vi "UPS_Monitor.vi"() -> ()   [LabVIEW 2023]
doc: "This is the Main VI that performs the UPS and capture data from DAQ and simulate the UPS"
uses:
  Controls/Acquired_Datactl_Display.ctl
  Controls/Queue_Operation_Select.ctl
  Controls/UPS_Data.ctl
  Controls/Acquired_Data.ctl
  Controls/State_and_Data.ctl
  Controls/Notifier_Operation_Select.ctl
  Controls/File_Operation_Select.ctl
  Controls/Error_Data.ctl
panel:
  out "Error_Out":errorcluster
  in  "Error_In":errorcluster
  in  "Tab Control":enum32{"PARAMETER", "DETAILS"}(tab)
  out "ACQUIRED_DATA":T1 {"Power_Consumption" scale=0.0..10.0; "Battery_Power" scale=0.0..100.0}
  out "Low_Power_Indicator":bool caption="Low Power Indicator"
  out "Waveform Graph":dbl[][](graph)
  in  "Record":bool
  in  "Stop":bool
  in  "Pause":bool
  in  "Start":bool
  # "UPS Monitor"
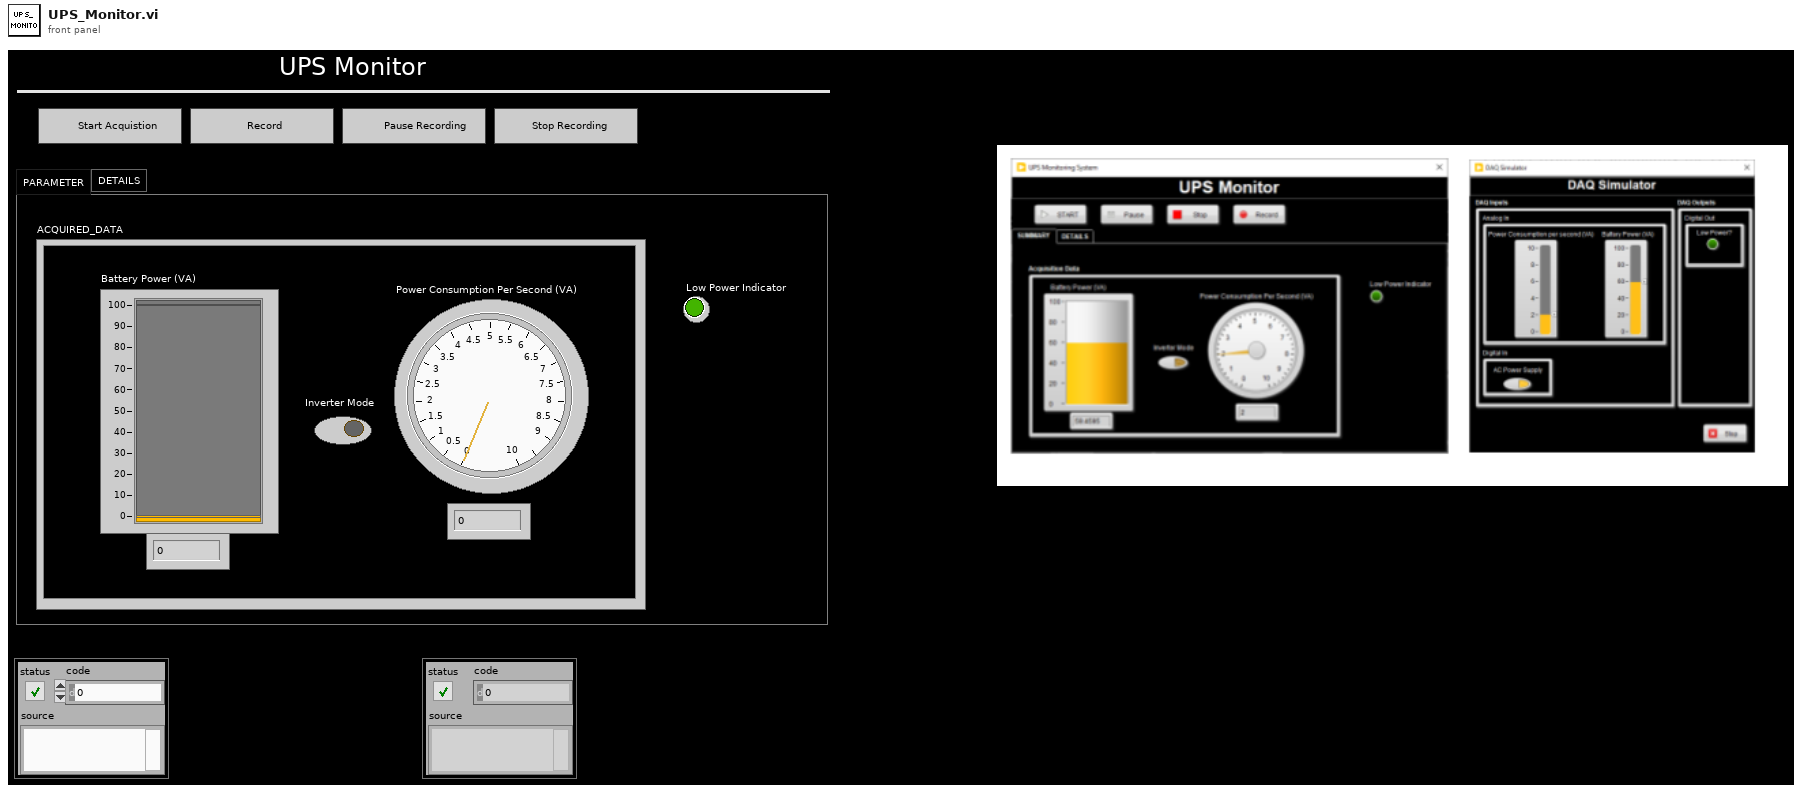
[diagram p1: front panel]
types:
  T1 = typedef "Acquired_Datactl_Display.ctl" = cluster{"Battery_Power":dbl, "Power_Consumption":dbl, "Inverter_Mode":bool}
  T2 = typedef "File_Operation_Select.ctl" = enum16{"Open", "Write", "Read", "Close"}
  T3 = typedef "Queue_Operation_Select.ctl" = enum16{"Obtain_Queue", "Enqueue", "Enqueue_First", "Enqueue_N", "Lossy_Enqueue", "Preview", "Queue_Status", "Dequeue", "Flush", "Release_Queue"}
  T4 = typedef "Notifier_Operation_Select.ctl" = enum16{"Obtain_Notifier", "Send_Notification", "Get_Notifier_Status", "Release_Notifier"}
  T5 = typedef "State_and_Data.ctl" = cluster{"State":string, "Data":variant}
  T6 = typedef "UPS_Data.ctl" = cluster{"ACQUIRED_DATA":T7, "Start":bool, "Pause":bool, "Record":bool, "Low_Power":bool, "Power_and_Power_Consumed":dbl[][], "State_and_Data_In":T5, "File_Path":path, "Application_Directory":path, "Record_Select":enum8{"Enabled", "Disabled", "Disabled and Grayed Out"}, "Stop_Select":enum8{"Enabled", "Disabled", "Disabled and Grayed Out"}}
  T7 = typedef "Acquired_Data.ctl" = cluster{"Battery_Power":dbl, "Power_Consumption":dbl, "Inverter_Mode":bool}
  T8 = enum8{"Enabled", "Disabled", "Disabled and Grayed Out"}
  T9 = typedef "Error_Data.ctl" = cluster{"Module_Name":string, "Error":errorcluster}
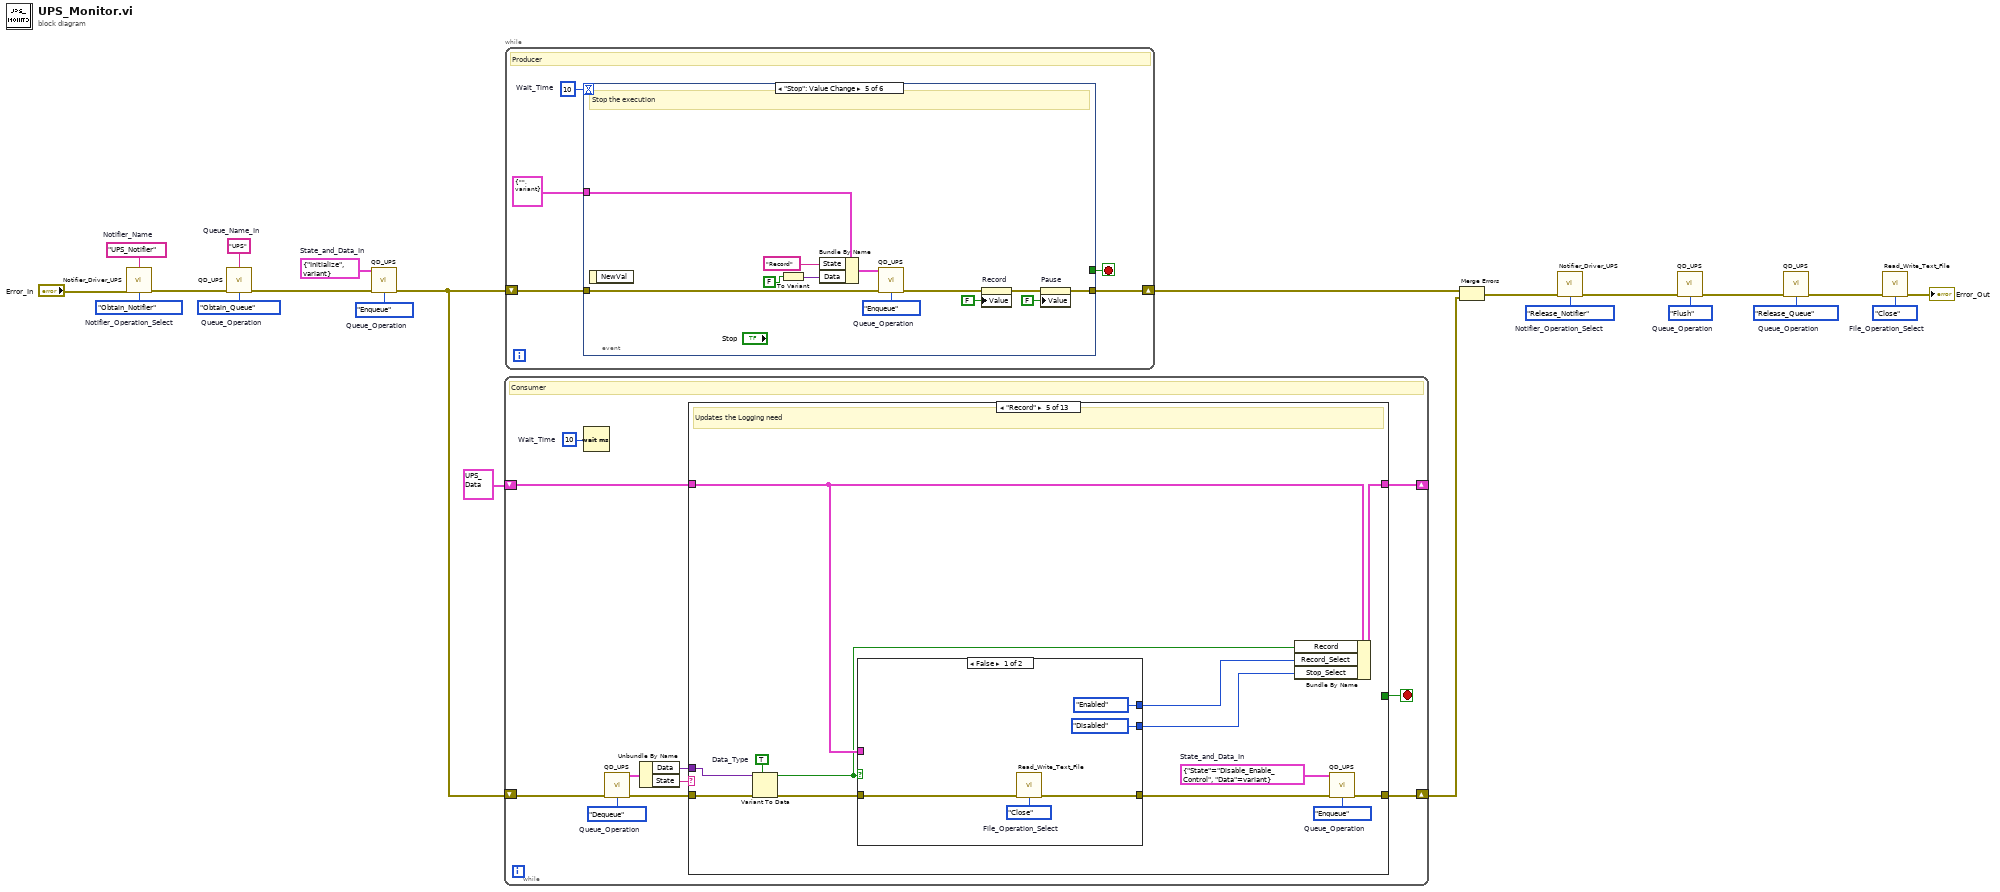
[diagram p0: block diagram]
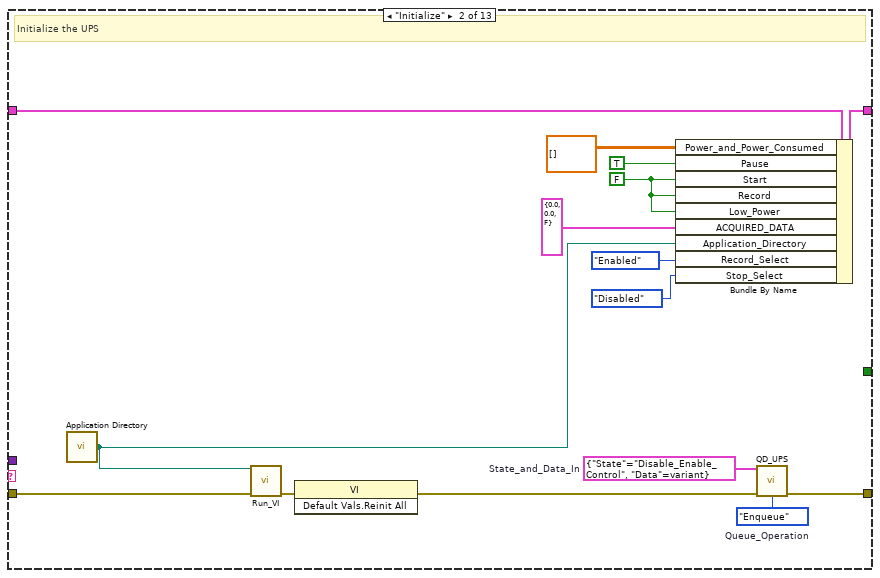
[diagram p3: hidden frame]
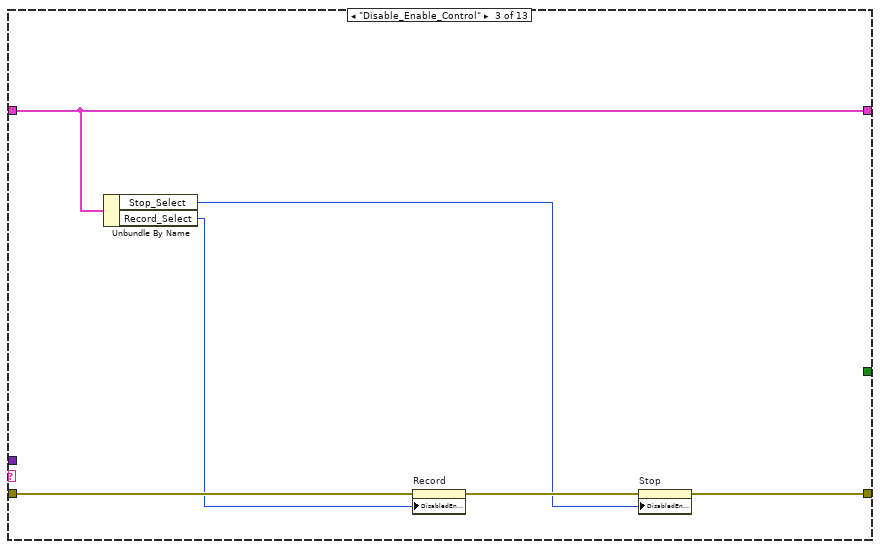
[diagram p4: hidden frame]
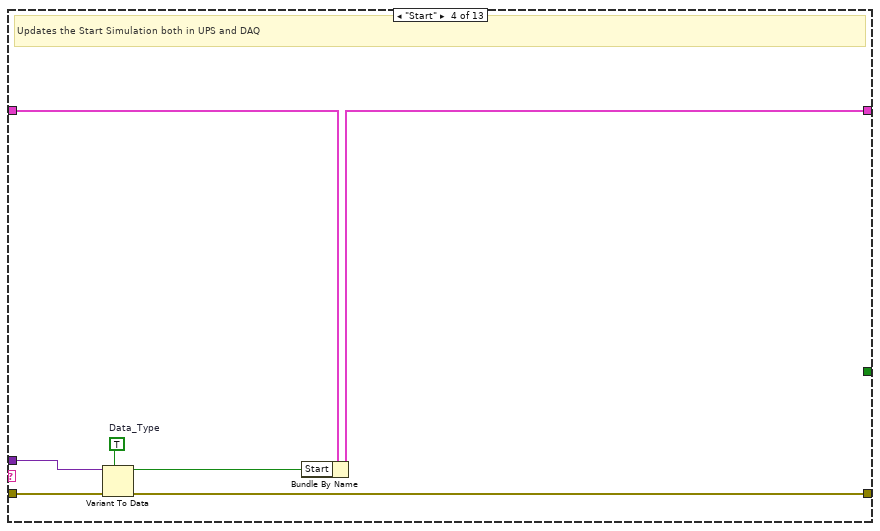
[diagram p5: hidden frame]
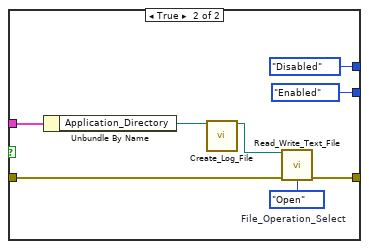
[diagram p6: hidden frame]
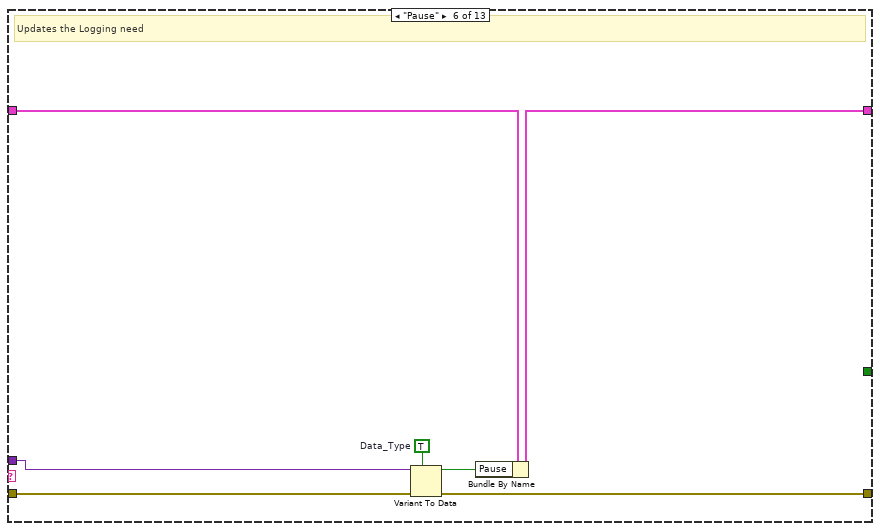
[diagram p7: hidden frame]
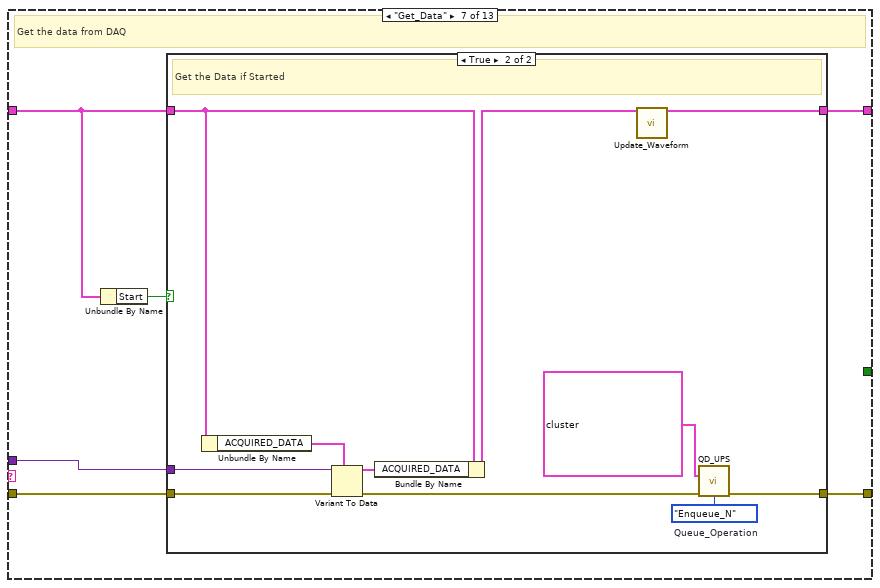
[diagram p8: hidden frame]
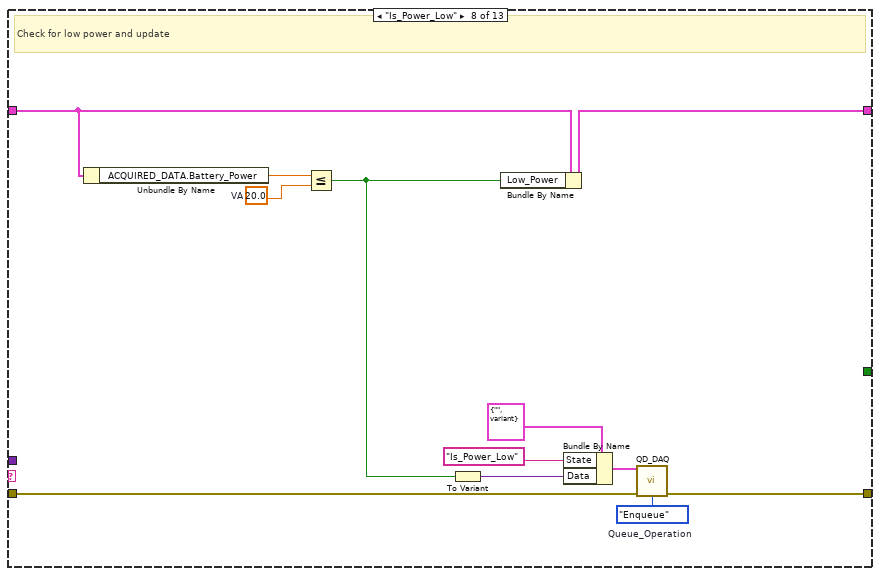
[diagram p10: hidden frame]
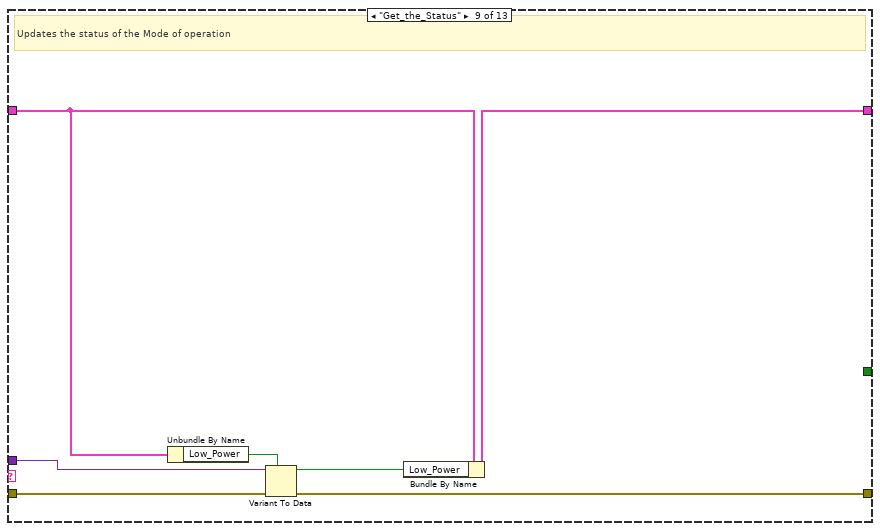
[diagram p11: hidden frame]
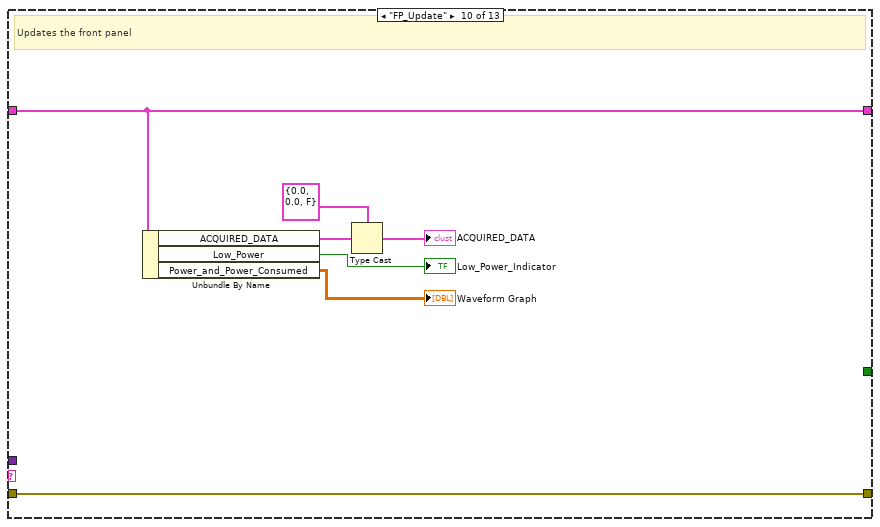
[diagram p12: hidden frame]
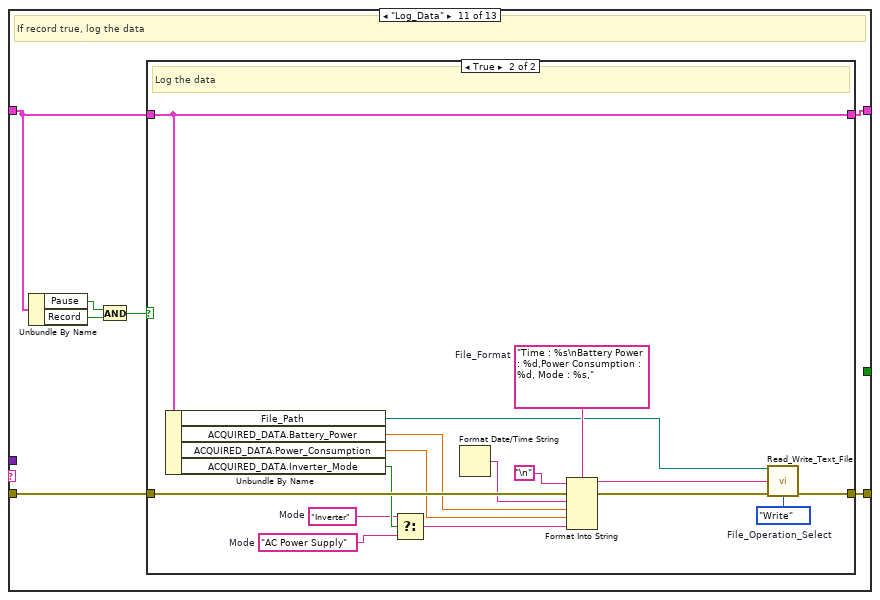
[diagram p13: hidden frame]
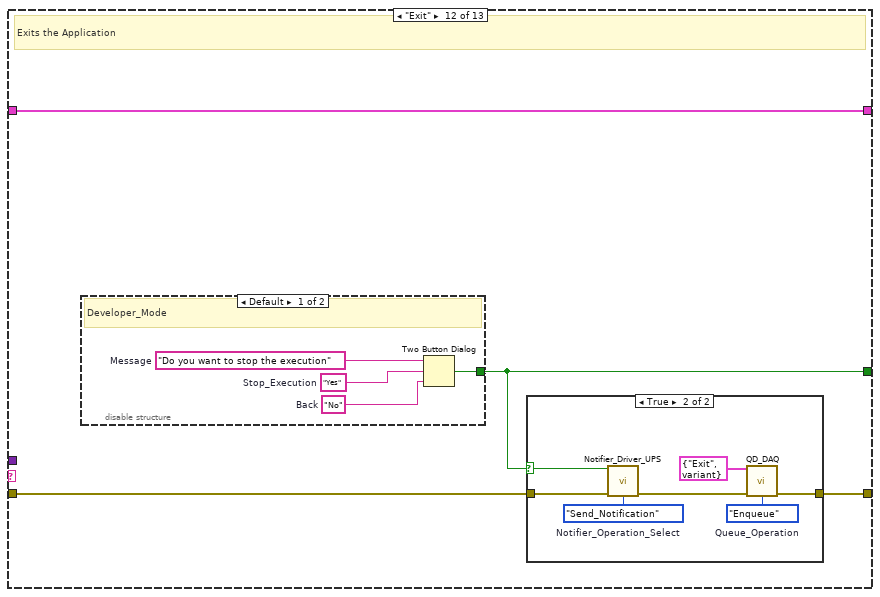
[diagram p15: hidden frame]
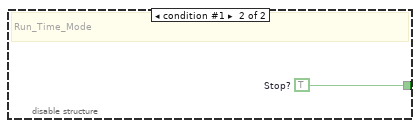
[diagram p17: hidden frame]
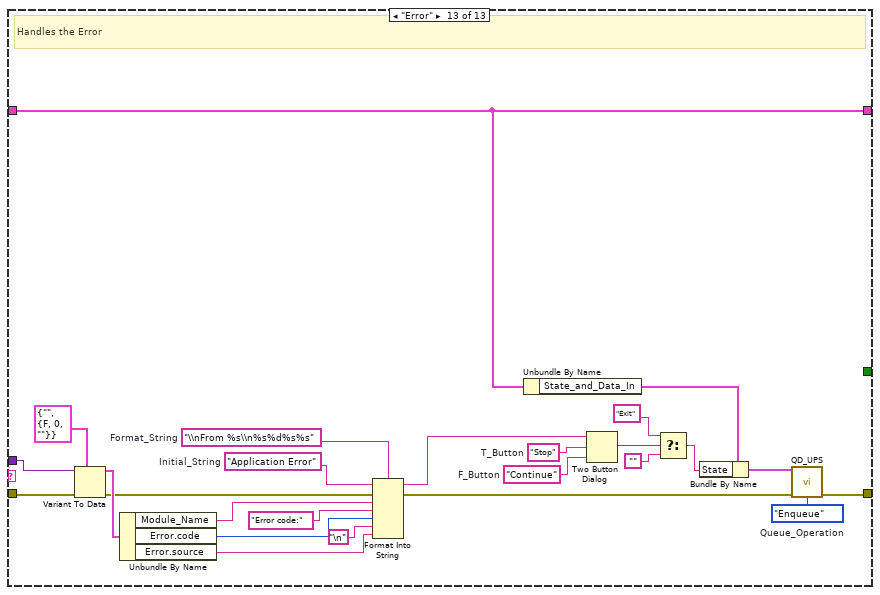
[diagram p18: hidden frame]
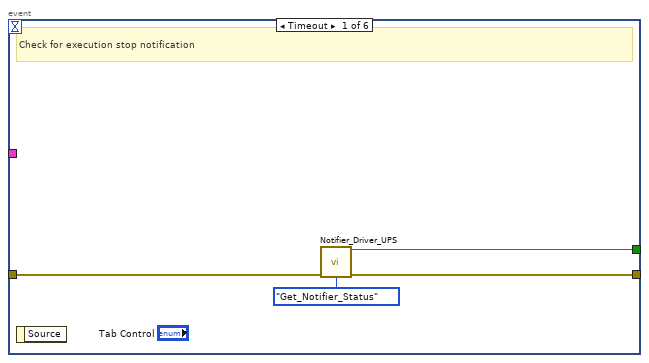
[diagram p19: hidden frame]
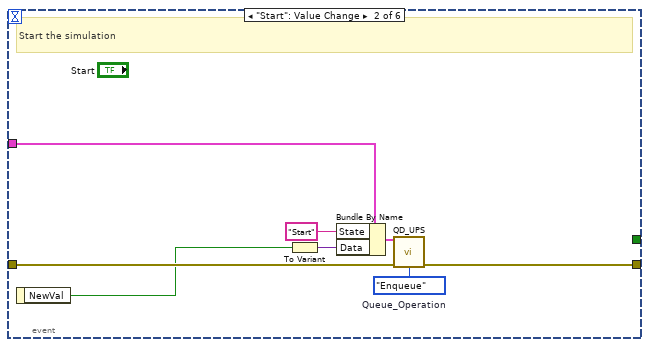
[diagram p20: hidden frame]
diagram:
  w7 = File_Operation_Select."Close"  # File_Operation_Select
  w8 = Queue_Operation_Select."Release_Queue"  # Queue_Operation
  w10 = Queue_Operation_Select."Flush"  # Queue_Operation
  w12 = Notifier_Operation_Select."Release_Notifier"  # Notifier_Operation_Select
  w14 = Notifier_Operation_Select."Obtain_Notifier"  # Notifier_Operation_Select
  w15 = "UPS_Notifier"  # Notifier_Name
  w17 = T5 {"State"="Initialize", "Data"=variant}  # State_and_Data_In
  w18 = Queue_Operation_Select."Enqueue"  # Queue_Operation
  w21 = "UPS"  # Queue_Name_In
  w22 = Queue_Operation_Select."Obtain_Queue"  # Queue_Operation
  n1 = call "Notifier_Driver_UPS.vi"("Notifier_Name"=w15, "Error_In"="Error_In", "Notifier_Operation_Select"=w14) -> ("Error_Out"=w16:errorcluster)  [unwired: 11 in, 1 out]
  n2 = call "QD_UPS.vi"("Queue_Name_In"=w21, "Error_In"=w16, "Queue_Operation"=w22) -> ("Error_Out"=w19:errorcluster)  [unwired: 11 in, 1 out]
  n3 = call "QD_UPS.vi"("State_and_Data_In"=w17, "Error_In"=w19, "Queue_Operation"=w18) -> ("Error_Out"=w2:errorcluster)  [unwired: 11 in, 1 out]
  n4 = while {
    shift-right: [w29] -> _
    shift-left: T6 {"ACQUIRED_DATA"={"Battery_Power"=0.0, "Power_Consumption"=0.0, "Inverter_Mode"=FALSE}, "Start"=TRUE, "Pause"=TRUE, "Record"=TRUE, "Low_Power"=TRUE, "Power_and_Power_Consumed"=[], "State_and_Data_In"={"State"="", "Data"=variant}, "File_Path"=path "", "Application_Directory"=path "", "Record_Select"=enum."Enabled", "Stop_Select"=enum."Enabled"} -> [w28]
    shift-right: [w24] -> w6
    shift-left: w2 -> [w33]
    stop <- w26 stop-if-true
    w23 = u32 10  # Wait_Time
    w25 = Queue_Operation_Select."Dequeue"  # Queue_Operation
    # "Consumer"
    n5 = Wait (ms)(milliseconds to wait=w23) -> ()  [unwired: 1 out]
    n6 = call "QD_UPS.vi"("Error_In"=w33, "Queue_Operation"=w25) -> ("State_and_Data_Out"=w31:T5, "Error_Out"=w32:errorcluster)  [unwired: 12 in]
    n7 = Unbundle By Name(w31) -> ("Data"=w27:variant, "State"=w30:string)
    n8 = case shown="\"Record\"" w30 {
      tunnel: w32 -> [w34 w43 w56 w63 w76 w95 w102 w127 w134 w141 w148 w169 w197]
      tunnel: [w35 w49 w53 w60 w75 w94 w99 w123 w133 w140 w146 w170 w196] -> w29
      tunnel: w28 -> [w35 w50 w53 w58 w72 w96 w98 w126 w129 w140 w145 w170 w196]
      tunnel: [w34 w40 w54 w57 w67 w93 w101 w122 w132 w141 w147 w168 w195] -> w24
      tunnel: w27 -> [_ _ _ w62 w74 w92 w100 _ w131 _ _ _ w192]
      tunnel: [_ _ _ _ _ _ _ _ _ _ _ w167 _] -> w26
      frame Default {
      }
      frame "Initialize" {
        w38 = T5 {"State"="Disable_Enable_Control", "Data"=variant}  # State_and_Data_In
        w39 = Queue_Operation_Select."Enqueue"  # Queue_Operation
        w37 = FALSE ("Start")
        # "Initialize the UPS"
        n9 = call <vilib>:"Application Directory.vi"() -> ("Application Directory"=w44:path)
        n10 = call "Run_VI.vi"("Application_Directory"=w44, "Error_In"=w43) -> ("Error_Out"=w46:errorcluster)  [unwired: 13 in]
        n11 = invoke class="VI" method="Default Vals.Reinit All"(error in=w46) -> (error out=w45:errorcluster)  [unwired: 2 in, 2 out]
        n12 = Bundle By Name(cluster=w50, "Power_and_Power_Consumed"=dbl[][] [], "Pause"=TRUE, "Start"=w37, "Record"=w37, "Low_Power"=w37, "ACQUIRED_DATA"=T7 {"Battery_Power"=0.0, "Power_Consumption"=0.0, "Inverter_Mode"=FALSE}, "Application_Directory"=w44, "Record_Select"=T8."Enabled", "Stop_Select"=T8."Disabled") -> (w49:T6)
        n13 = call "QD_UPS.vi"("State_and_Data_In"=w38, "Error_In"=w45, "Queue_Operation"=w39) -> ("Error_Out"=w40:errorcluster)  [unwired: 11 in, 1 out]
      }
      frame "Disable_Enable_Control" {
        n14 = Unbundle By Name(w53) -> ("Stop_Select"=w51:T8, "Record_Select"=w52:T8)
        n15 = property on="Record" class="Bool (strict)"(error in=w56, "DisabledEnum"=w52) -> (error out=w55:errorcluster)  [unwired: 1 in, 1 out]
        n16 = property on="Stop" class="Bool"(error in=w55, "DisabledEnum"=w51) -> (error out=w54:errorcluster)  [unwired: 1 in, 1 out]
      }
      frame "Start" {
        w61 = TRUE  # Data_Type
        # "Updates the Start Simulation both in UPS and DAQ"
        n17 = Variant To Data(error in=w63, type=w61, Variant=w62) -> (data=w59:bool, error out=w57:errorcluster)
        n18 = Bundle By Name(cluster=w58, "Start"=w59) -> (w60:T6)
      }
      frame "Record" {
        w66 = T5 {"State"="Disable_Enable_Control", "Data"=variant}  # State_and_Data_In
        w69 = Queue_Operation_Select."Enqueue"  # Queue_Operation
        w73 = TRUE  # Data_Type
        # "Updates the Logging need"
        n19 = Variant To Data(error in=w76, type=w73, Variant=w74) -> (data=w70:bool, error out=w71:errorcluster)
        n20 = case shown="False" w70 {
          tunnel: w72 -> [_ w89]
          tunnel: [w80 w88] -> w68
          tunnel: w71 -> [w81 w85]
          tunnel: [T8."Disabled" ("Stop_Select") T8."Enabled" ("Stop_Select")] -> w65
          tunnel: [T8."Enabled" ("Record_Select") T8."Disabled" ("Record_Select")] -> w64
          frame False {
            w79 = File_Operation_Select."Close"  # File_Operation_Select
            n21 = call "Read_Write_Text_File.vi"("Error_In"=w81, "File_Operation_Select"=w79) -> ("Error_Out"=w80:errorcluster)  [unwired: 12 in, 1 out]
          }
          frame True {
            w87 = File_Operation_Select."Open"  # File_Operation_Select
            n22 = Unbundle By Name(w89) -> ("Application_Directory"=w84:path)
            n23 = call "Create_Log_File.vi"("Application_Directory"=w84) -> ("New_File_Path"=w86:path)  [unwired: 14 in]
            n24 = call "Read_Write_Text_File.vi"("File_Path"=w86, "Error_In"=w85, "File_Operation_Select"=w87) -> ("Error_Out"=w88:errorcluster)  [unwired: 11 in, 1 out]
          }
        }
        n25 = Bundle By Name(cluster=w72, "Record"=w70, "Record_Select"=w64, "Stop_Select"=w65) -> (w75:T6)
        n26 = call "QD_UPS.vi"("State_and_Data_In"=w66, "Error_In"=w68, "Queue_Operation"=w69) -> ("Error_Out"=w67:errorcluster)  [unwired: 11 in, 1 out]
      }
      frame "Pause" {
        w91 = TRUE  # Data_Type
        # "Updates the Logging need"
        n27 = Variant To Data(error in=w95, type=w91, Variant=w92) -> (data=w90:bool, error out=w93:errorcluster)
        n28 = Bundle By Name(cluster=w96, "Pause"=w90) -> (w94:T6)
      }
      frame "Get_Data" {
        # "Get the data from DAQ"
        n29 = Unbundle By Name(w98) -> ("Start"=w97:bool)
        n30 = case shown="True" w97 {
          tunnel: w102 -> [w103 w115]
          tunnel: [w103 w108] -> w101
          tunnel: w100 -> [_ w113]
          tunnel: w98 -> [w104 w112]
          tunnel: [w104 w105] -> w99
          frame False {
          }
          frame True {
            w107 = Queue_Operation_Select."Enqueue_N"  # Queue_Operation
            # "Get the Data if Started"
            n31 = Unbundle By Name(w112) -> ("ACQUIRED_DATA"=w111:T7)
            n32 = Variant To Data(error in=w115, type=w111, Variant=w113) -> (data=w109:T7, error out=w114:errorcluster)
            n33 = Bundle By Name(cluster=w112, "ACQUIRED_DATA"=w109) -> (w110:T6)
            n34 = call "Update_Waveform.vi"("Data"=w110) -> ("Update_Data"=w105:T6)  [unwired: 14 in]
            n35 = call "QD_UPS.vi"("State_and_Data_N_In"=T5[] [{"State"="Is_Power_Low", "Data"=variant}, {"State"="FP_Update", "Data"=variant}, {"State"="Log_Data", "Data"=variant}], "Error_In"=w114, "Queue_Operation"=w107) -> ("Error_Out"=w108:errorcluster)  [unwired: 11 in, 1 out]
          }
        }
      }
      frame "Is_Power_Low" {
        w120 = Queue_Operation_Select."Enqueue"  # Queue_Operation
        w124 = 20.0  # VA
        # "Check for low power and update"
        n36 = Unbundle By Name(w126) -> ("ACQUIRED_DATA.Battery_Power"=w125:dbl)
        n37 = Less Or Equal?(x=w125, y=w124) -> (x <= y?=w121:bool)
        n38 = To Variant(anything=w121) -> (Variant=w116:variant)
        n39 = Bundle By Name(cluster=w126, "Low_Power"=w121) -> (w123:T6)
        n40 = Bundle By Name(cluster=T5 {"State"="", "Data"=variant} ("Data_In"), "State"="Is_Power_Low", "Data"=w116) -> (w117:T5)
        n41 = call "QD_DAQ.vi"("State_and_Data_In"=w117, "Error_In"=w127, "Queue_Operation"=w120) -> ("Error_Out"=w122:errorcluster)  [unwired: 11 in, 1 out]
      }
      frame "Get_the_Status" {
        # "Updates the status of the Mode of operation"
        n42 = Unbundle By Name(w129) -> ("Low_Power"=w128:bool)
        n43 = Variant To Data(error in=w134, type=w128, Variant=w131) -> (data=w130:bool, error out=w132:errorcluster)
        n44 = Bundle By Name(cluster=w129, "Low_Power"=w130) -> (w133:T6)
      }
      frame "FP_Update" {
        # "Updates the front panel"
        n45 = Unbundle By Name(w140) -> ("ACQUIRED_DATA"=w139:T7, "Low_Power"=→"Low_Power_Indicator":bool, "Power_and_Power_Consumed"=→"Waveform Graph":dbl[][])
        n46 = Type Cast(type=T1 {"Battery_Power"=0.0, "Power_Consumption"=0.0, "Inverter_Mode"=FALSE} ("ACQUIRED_DATA"), x=w139) -> (*(type *) &x=→"ACQUIRED_DATA":T1)
      }
      frame "Log_Data" {
        # "If record true, log the data"
        n47 = Unbundle By Name(w145) -> ("Pause"=w142:bool, "Record"=w144:bool)
        n48 = And(x=w142, y=w144) -> (x .and. y?=w143:bool)
        n49 = case shown="True" w143 {
          tunnel: w145 -> [w150 w159]
          tunnel: w148 -> [w149 w166]
          tunnel: [w149 w165] -> w147
          tunnel: [w150 w159] -> w146
          frame False {
          }
          frame True {
            w153 = "AC Power Supply"  # Mode
            w154 = "Inverter"  # Mode
            w161 = "Time : %s\nBattery Power : %d,Power Consumption : %d, Mode : %s,"  # File_Format
            w164 = File_Operation_Select."Write"  # File_Operation_Select
            # "Log the data"
            n50 = Unbundle By Name(w159) -> ("File_Path"=w157:path, "ACQUIRED_DATA.Battery_Power"=w152:dbl, "ACQUIRED_DATA.Power_Consumption"=w160:dbl, "ACQUIRED_DATA.Inverter_Mode"=w156:bool)
            n51 = Select(t=w154, s=w156, f=w153) -> (s? t:f=w155:string)
            n52 = Format Date/Time String() -> (date/time string=w151:string)  [unwired: 3 in]
            n53 = Format Into String(format string=w161, initial string="\n", error in=w166, w151, w152, w160, w155) -> (resulting string=w162:string, error out=w163:errorcluster)
            n54 = call "Read_Write_Text_File.vi"("File_Path"=w157, "Data"=w162, "Error_In"=w163, "File_Operation_Select"=w164) -> ("Error_Out"=w165:errorcluster)  [unwired: 10 in, 1 out]
          }
        }
      }
      frame "Exit" {
        # "Exits the Application"
        n55 = disable-structure shown="Default" {
          disable-tunnel: [w179 w183] -> w167
          frame condition #0 (active) {
            w180 = "No"  # Back
            w181 = "Yes"  # Stop_Execution
            w182 = "Do you want to stop the execution"  # Message
            # "Developer_Mode"
            n56 = Two Button Dialog(message=w182, 1:w180, 2:w181) -> (T button?=w179:bool)
          }
          frame condition #1 {
            w183 = TRUE  # Stop?
            # "Run_Time_Mode"
          }
        }
        n57 = case shown="True" w167 {
          selector: w167 -> [_ w172]
          tunnel: w169 -> [w171 w178]
          tunnel: [w171 w177] -> w168
          frame False {
          }
          frame True {
            w173 = Notifier_Operation_Select."Send_Notification"  # Notifier_Operation_Select
            w176 = Queue_Operation_Select."Enqueue"  # Queue_Operation
            n58 = call "Notifier_Driver_UPS.vi"("Notification"=w172, "Error_In"=w178, "Notifier_Operation_Select"=w173) -> ("Error_Out"=w174:errorcluster)  [unwired: 11 in, 1 out]
            n59 = call "QD_DAQ.vi"("State_and_Data_In"=T5 {"State"="Exit", "Data"=variant}, "Error_In"=w174, "Queue_Operation"=w176) -> ("Error_Out"=w177:errorcluster)  [unwired: 11 in, 1 out]
          }
        }
      }
      frame "Error" {
        w193 = Queue_Operation_Select."Enqueue"  # Queue_Operation
        w204 = "\\nFrom %s\\n%s%d%s%s"  # Format_String
        w205 = "Application Error"  # Initial_String
        w206 = "Stop"  # T_Button
        w207 = "Continue"  # F_Button
        # "Handles the Error"
        n60 = Variant To Data(error in=w197, type=T9 {"Module_Name"="", "Error"={"status"=FALSE, "code"=0, "source"=""}} ("Error_Data"), Variant=w192) -> (data=w190:T9, error out=w185:errorcluster)
        n61 = Unbundle By Name(w190) -> ("Module_Name"=w189:string, "Error.code"=w188:i32, "Error.source"=w186:string)
        n62 = Format Into String(format string=w204, initial string=w205, error in=w185, w189, "Error code:" ("input 2"), w188, "\n", w186) -> (resulting string=w208:string, error out=w198:errorcluster)
        n63 = Unbundle By Name(w196) -> ("State_and_Data_In"=w199:T5)
        n64 = Two Button Dialog(message=w208, 1:w207, 2:w206) -> (T button?=w202:bool)
        n65 = Select(t="Exit" ("State"), s=w202, f="") -> (s? t:f=w200:string)
        n66 = Bundle By Name(cluster=w199, "State"=w200) -> (w194:T5)
        n67 = call "QD_UPS.vi"("State_and_Data_In"=w194, "Error_In"=w198, "Queue_Operation"=w193) -> ("Error_Out"=w195:errorcluster)  [unwired: 11 in, 1 out]
      }
    }
  }
  n68 = while {
    shift-right: [w209] -> w5
    shift-left: w2 -> [w213]
    stop <- w212 stop-if-true
    w211 = 10  # Wait_Time
    # "Producer"
    n69 = event shown="[4] \"Stop\": Value Change" {
      selector: _ -> [_ _ _ _ _ _]
      dyn-events: _ -> [_ _ _ _ _ _]
      timeout: w211 -> [_ _ _ _ _ _]
      tunnel: w213 -> [w217 w219 w227 w239 w251 w259]
      tunnel: [w216 w220 w228 w235 w244 w258] -> w209
      tunnel: [w214 _ _ _ _ _] -> w212
      tunnel: T5 {"State"="", "Data"=variant} ("State_and_Data_In") -> [_ w225 w234 w237 w249 w256]
      event Timeout {
        # "Check for execution stop notification"
        n70 = event-data() -> ()  [unwired: 1 in, 1 out]
        n71 = call "Notifier_Driver_UPS.vi"("Error_In"=w217, "Notifier_Operation_Select"=Notifier_Operation_Select."Get_Notifier_Status") -> ("Latest_Notification"=w214:bool, "Error_Out"=w216:errorcluster)  [unwired: 12 in]
      }
      event "Start": Value Change {
        w224 = Queue_Operation_Select."Enqueue"  # Queue_Operation
        # "Start the simulation"
        n72 = event-data() -> ("NewVal"=w218:bool)  [unwired: 1 in]
        n73 = To Variant(anything=w218) -> (Variant=w222:variant)
        n74 = Bundle By Name(cluster=w225, "State"="Start", "Data"=w222) -> (w223:T5)
        n75 = call "QD_UPS.vi"("State_and_Data_In"=w223, "Error_In"=w219, "Queue_Operation"=w224) -> ("Error_Out"=w220:errorcluster)  [unwired: 11 in, 1 out]
      }
      event "Pause": Value Change {
        w230 = Queue_Operation_Select."Enqueue"  # Queue_Operation
        # "Pause the simulation"
        n76 = event-data() -> ("NewVal"=w233:bool)  [unwired: 1 in]
        n77 = Not(x=w233) -> (.not. x?=w226:bool)
        n78 = To Variant(anything=w226) -> (Variant=w231:variant)
        n79 = Bundle By Name(cluster=w234, "State"="Pause", "Data"=w231) -> (w232:T5)
        n80 = call "QD_UPS.vi"("State_and_Data_In"=w232, "Error_In"=w227, "Queue_Operation"=w230) -> ("Error_Out"=w228:errorcluster)  [unwired: 11 in, 1 out]
      }
      event "Record": Value Change {
        w242 = Queue_Operation_Select."Enqueue"  # Queue_Operation
        # "Log the data into the file"
        n81 = event-data() -> ()  [unwired: 1 in, 1 out]
        n82 = To Variant(anything=TRUE ("Record")) -> (Variant=w240:variant)
        n83 = Bundle By Name(cluster=w237, "State"="Record", "Data"=w240) -> (w241:T5)
        n84 = call "QD_UPS.vi"("State_and_Data_In"=w241, "Error_In"=w239, "Queue_Operation"=w242) -> ("Error_Out"=w235:errorcluster)  [unwired: 11 in, 1 out]
      }
      event "Stop": Value Change {
        w254 = Queue_Operation_Select."Enqueue"  # Queue_Operation
        # "Stop the execution"
        n85 = event-data() -> ()  [unwired: 1 in, 1 out]
        n86 = To Variant(anything=FALSE ("Stop")) -> (Variant=w252:variant)
        n87 = Bundle By Name(cluster=w249, "State"="Record", "Data"=w252) -> (w253:T5)
        n88 = call "QD_UPS.vi"("State_and_Data_In"=w253, "Error_In"=w251, "Queue_Operation"=w254) -> ("Error_Out"=w247:errorcluster)  [unwired: 11 in, 1 out]
        n89 = property on="Record" class="Bool (strict)"(error in=w247, "Value"=FALSE ("Record")) -> (error out=w246:errorcluster)  [unwired: 1 in, 1 out]
        n90 = property on="Pause" class="Bool (strict)"(error in=w246, "Value"=FALSE ("Pause")) -> (error out=w244:errorcluster)  [unwired: 1 in, 1 out]
      }
      event Panel Close? {
        w257 = Queue_Operation_Select."Enqueue"  # Queue_Operation
        # "Stop the execution"
        n91 = event-data() -> ()  [unwired: 1 in, 4 out]
        n92 = Bundle By Name(cluster=w256, "State"="Exit") -> (w260:T5)
        n93 = call "QD_UPS.vi"("State_and_Data_In"=w260, "Error_In"=w259, "Queue_Operation"=w257) -> ("Error_Out"=w258:errorcluster)  [unwired: 11 in, 1 out]
        n94 = event-data("Discard?"=TRUE) -> ()  [unwired: 1 in, 1 out]
      }
    }
  }
  n95 = Merge Errors(w5, w6) -> (w4:errorcluster)
  n96 = call "Notifier_Driver_UPS.vi"("Error_In"=w4, "Notifier_Operation_Select"=w12) -> ("Error_Out"=w13:errorcluster)  [unwired: 12 in, 1 out]
  n97 = call "QD_UPS.vi"("Error_In"=w13, "Queue_Operation"=w10) -> ("Error_Out"=w11:errorcluster)  [unwired: 12 in, 1 out]
  n98 = call "QD_UPS.vi"("Error_In"=w11, "Queue_Operation"=w8) -> ("Error_Out"=w9:errorcluster)  [unwired: 12 in, 1 out]
  n99 = call "Read_Write_Text_File.vi"("Error_In"=w9, "File_Operation_Select"=w7) -> ("Error_Out"=→"Error_Out":errorcluster)  [unwired: 12 in, 1 out]
